vi "20170425-lecture4-1 string match regexp patterns.vi"() -> ()   [LabVIEW 2014]
uses:
  <vilib>/regexp/Match Regular Expression.xnode
panel:
  out "submatch 4":string
  out "submatch 3":string
  out "submatch 2":string
  out "submatch 1":string
  in  "input string":string="Volts dc-1.2312; "
  in  "regular expression":string="([Vv][Oo][Ll][Tt][Ss]|[Aa][Mm][Pp][Ee][Rr])\\s+([AaDd][cC])([\\s+-])([0-9\\.]+).*"
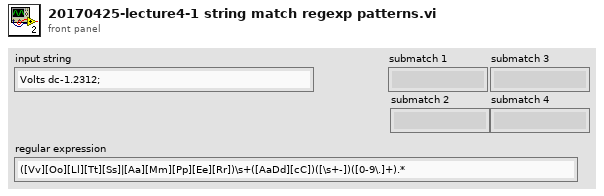
[diagram p1: front panel]
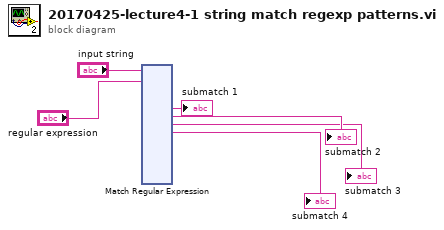
[diagram p0: block diagram]
diagram:
  n1 = xnode "Match Regular Expression"("input string"="input string", "regular expression"="regular expression") -> ("submatch 1"=→"submatch 1":string, "submatch 2"=→"submatch 2":string, "submatch 3"=→"submatch 3":string, "submatch 4"=→"submatch 4":string)  [unwired: 4 in, 11 out]
